vi "validate configuration.vi"(8 "error in":errorcluster, 11 "asynchronous execution component configuration in":refnum<class "asynchronous execution module configuration.lvclass">) -> (0 "error out":errorcluster, 3 "asynchronous execution component configuration out":refnum<class "asynchronous execution module configuration.lvclass">)   [LabVIEW 2013, in "asynchronous execution module configuration.lvclass"]
doc: "This function performs validation of the configuration. This function should be safe to call at any point and should not rely on anything in the runtime environment."
uses:
  asynchronous execution module configuration.lvclass
  <vilib>/NI/Tag Bus Module Framework/module configuration/TBM module configuration.lvclass
  asynchronous execution module configuration.lvclass/asynchronous execution module configuration.ctl
  <vilib>/NI/Tag Bus Module Framework/root configuration/TBM configuration.lvclass
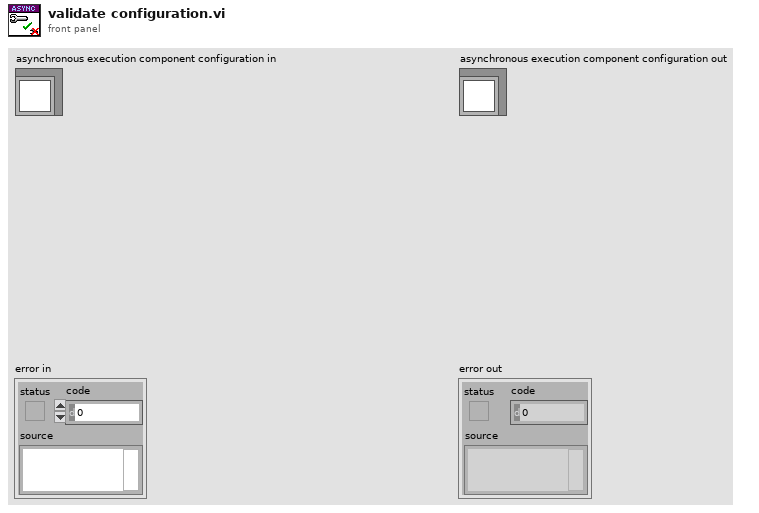
[diagram p1: front panel]
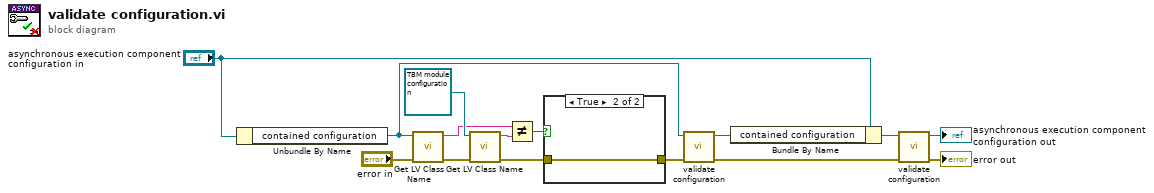
[diagram p0: block diagram]
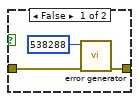
[diagram p2: hidden frame]
diagram:
  n1 = Unbundle By Name("asynchronous execution component configuration in") -> ("contained configuration"=w15:refnum<class "TBM module configuration.lvclass">)
  n2 = call <vilib>:"Get LV Class Name.vi"("error in (no error)"="error in", "object"=w15) -> ("error out"=w10:errorcluster, "class name"=w8:string)  [unwired: 8 in]
  n3 = call <vilib>:"Get LV Class Name.vi"("error in (no error)"=w10, "object"=refnum<class "TBM module configuration.lvclass"> refnum ("component configuration")) -> ("error out"=w5:errorcluster, "class name"=w7:string)  [unwired: 8 in]
  n4 = Not Equal?(x=w8, y=w7) -> (x != y?=w6:bool)
  n5 = case shown="True" w6 {
    tunnel: w5 -> [w17 w19]
    tunnel: [w16 w19] -> w4
    frame False {
      n6 = call <vilib>:"error generator.vi"("error in"=w17, "error code (0)"=538288) -> ("error out"=w16:errorcluster)  [unwired: 9 in]
    }
    frame True {
    }
  }
  n7 = call-dynamic "validate configuration.vi"("error in"=w4, "configuration in"=w15) -> ("error out"=w12:errorcluster, "configuration out"=w13:refnum<class "TBM module configuration.lvclass">)  [unwired: 8 in]
  n8 = Bundle By Name(cluster="asynchronous execution component configuration in", "contained configuration"=w13) -> (w2:refnum<class "asynchronous execution module configuration.lvclass">)
  n9 = call-parent "validate configuration.vi"("error in"=w12, "configuration in"=w2) -> ("error out"=→"error out":errorcluster, "configuration out"=→"asynchronous execution component configuration out":refnum<class "asynchronous execution module configuration.lvclass">)  [unwired: 8 in]
